vi "Set Up Tree Browser.vi"(7 "Tree Ref":T1, 11 "Item Ref in":T2 format="%.0x") -> ()   [LabVIEW 2019, in "Software Multi-Plex System Explorer.lvlib"]
uses:
  Software Multi-Plex System Explorer.lvlib
  <vilib>/NI VeriStand/Custom Device API/Custom Device Item Ref.ctl
  <vilib>/NI VeriStand/UI Controls/Tree and Alias Browser/Tree Alias Browser Display.ctl
  NationalInstruments.VeriStand.SystemStorageUI
  <vilib>/NI VeriStand/Custom Device Tools/Custom Device Utility Library/Custom Device Utility Library.lvlib
  <vilib>/NI VeriStand/Custom Device API/Custom Device API.lvlib
  <vilib>/NI VeriStand/UI Controls/Tree and Alias Browser/NI_VS UI Tree Alias Browser.lvlib
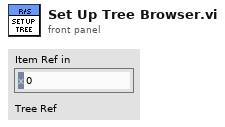
[diagram p1: front panel]
types:
  T1 = typedef "NI_VS UI Tree Alias Browser.lvlib/Tree Alias Browser Display.ctl" = refnum<k24>
  T2 = typedef "Custom Device API.lvlib/Custom Device Item Ref.ctl" = u64
  T3 = typedef "Custom Device API.lvlib/Custom Device Pointer.ctl" = refnum<k24>
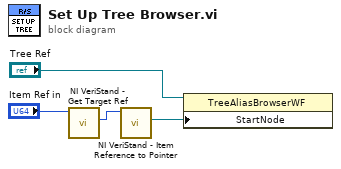
[diagram p0: block diagram]
diagram:
  n1 = call <vilib>:"NI VeriStand - Get Target Ref.vi"("Item Ref in"="Item Ref in") -> ("Target Ref"=w4:T2)  [unwired: 7 in, 3 out]
  n2 = call <vilib>:"NI VeriStand - Item Reference to Pointer.vi"("Item Ref in"=w4) -> ("Node Pointer"=w3:T3)  [unwired: 7 in, 3 out]
  n3 = property class="TreeAliasBrowserWF"(reference="Tree Ref", "StartNode"=w3) -> ()  [unwired: 1 in, 2 out]
